vi "Limit AO Amplitude.vi"(8 "error in (no error)":errorcluster, 11 "Instrument.DAQ":refnum<class "Instrument.DAQ.lvclass">) -> (0 "error out":errorcluster, 3 "Instrument.DAQ out":refnum<class "Instrument.DAQ.lvclass">)   [LabVIEW 2019, in "Instrument.Lockin.lvlib" / "Instrument.DAQ.lvclass"]
uses:
  Instrument.DAQ.lvclass
  Instrument.DAQ.lvclass/Instrument.DAQ.ctl
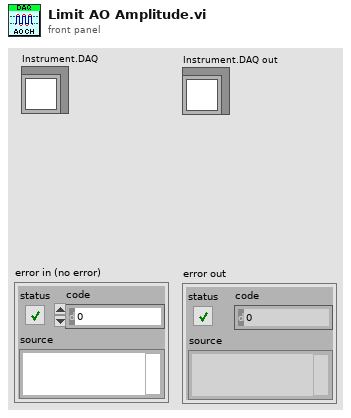
[diagram p1: front panel]
types:
  T1 = typedef "Instrument.Lockin.lvlib/Instrument.DAQ.lvclass/AO.Channel--Cluster--Array.ctl" = T2[]
  T2 = typedef "Instrument.Lockin.lvlib/Instrument.DAQ.lvclass/AO.Channel--Cluster.ctl" = cluster{"Enable?":bool, "Channel":i32, "Amplitude":dbl, "Offset":dbl, "Frequency":dbl, "Phase":dbl, "Function":T3, "Sweeping?":bool}
  T3 = typedef "Instrument.Lockin.lvlib/Instrument.DAQ.lvclass/AO.Channel.Function--Enum.ctl" = enum16{"Sine", "Triangle", "Square"}
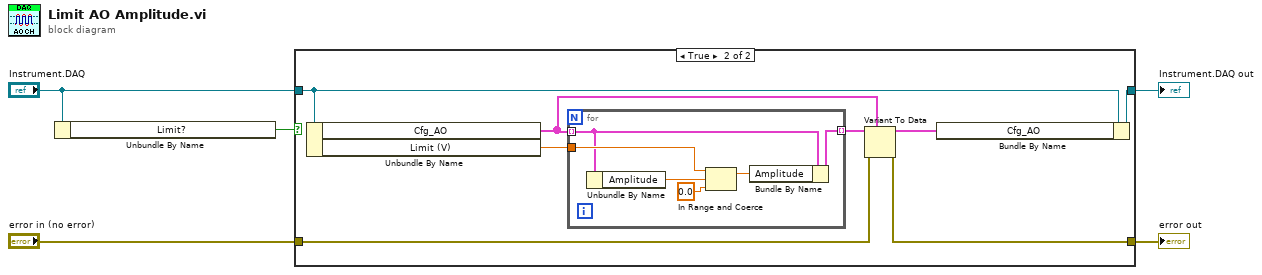
[diagram p0: block diagram]
diagram:
  n1 = Unbundle By Name("Instrument.DAQ") -> ("Limit?"=w1:bool)
  n2 = case shown="True" w1 {
    tunnel: [w6 w15] -> w5
    tunnel: "Instrument.DAQ" -> [w6 w14]
    tunnel: "error in (no error)" -> [w7 w10]
    tunnel: [w7 w11] -> w3
    frame False {
    }
    frame True {
      n3 = Unbundle By Name(w14) -> ("Cfg_AO"=w9:T1, "Limit (V)"=w8:dbl)
      n4 = for {
        tunnel: w9 -> [w18] mode=indexing
        tunnel: w8 -> [w19]
        tunnel: [w16] -> w13 mode=indexing
        n5 = Unbundle By Name(w18) -> ("Amplitude"=w20:dbl)
        n6 = In Range and Coerce(upper limit=w19, x=w20, lower limit=0.0) -> (coerced(x)=w17:dbl)  [unwired: 1 out]
        n7 = Bundle By Name(cluster=w18, "Amplitude"=w17) -> (w16:T2)
      }
      n8 = Variant To Data(error in=w10, type=w9, Variant=w13) -> (data=w12:T1, error out=w11:errorcluster)
      n9 = Bundle By Name(cluster=w14, "Cfg_AO"=w12) -> (w15:refnum<class "Instrument.DAQ.lvclass">)
    }
  }
  "Instrument.DAQ out" <- w5
  "error out" <- w3
